vi "ROI Stand alone - get previous Zstack protocol.vi"(8 "error in (no error)":errorcluster, 11 "path":path) -> (0 "error out":errorcluster, 1 "Protocol":string, 2 "Frame Size":T1=200 items=["100X100"=100, "128X128"=128, "200X200"=200, "256X256"=256, "512X512"=512, "1024x1024"=1024, "2048x2048"=2048], 3 "field of view":dbl, 5 "zoom":dbl)   [LabVIEW 2020]
uses:
  Typedefs/Frame Size.ctl
  Visualisation/Functional Imaging Viewer/SubVIs/Experiment header interface/Typedefs/Header file actions.ctl
  Visualisation/Functional Imaging Viewer/SubVIs/Experiment header interface/Typedefs/Header file sections.ctl
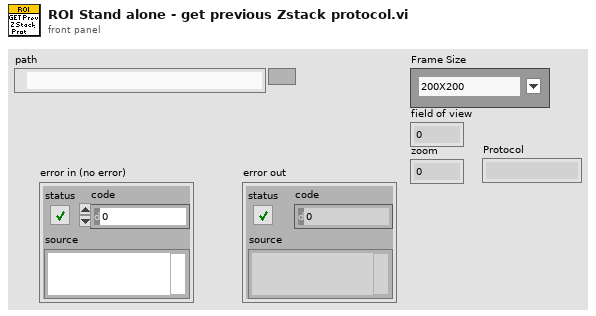
[diagram p1: front panel]
types:
  T1 = typedef "Frame Size.ctl" = u16
  T2 = typedef "Header file sections.ctl" = enum16{"ALL SECTIONS", "LOGIN", "GLOBAL PARAMETERS", "CALIBRATION DATA", "IMAGING MODES", "TIME SERIES", "MOTOR Z-STACK", "AOL Z-STACK", "FUNCTIONAL IMAGING", "VOLUME IMAGING", "MOVEMENT CORRECTION", "CALIBRATION", "STATISTICS", "BIOLOGY INFORMATION"}
  T3 = typedef "Header file actions.ctl" = enum16{"Create", "Open", "Read All", "Read Section", "Write All", "Write Section", "Close"}
  T4 = typedef "Header parameters cluster-ALL.ctl" = cluster{"LOGIN":T5, "GLOBAL PARAMETERS":T6, "IMAGING MODES":T8, "TIME SERIES":T9, "MOTOR Z-STACK ":T11, "AOL Z-STACK":T12, "FUNCTIONAL IMAGING":T13, "VOLUME IMAGING":T13, "MOVEMENT CORRECTION":T17, "CALIBRATION":T19, "STATISTICS":T20, "BIOLOGY INFORMATION":T21, "Calibration Data":T22}
  T5 = typedef "Header params -Login.ctl" = cluster{"User":string, "Profile":string, "Software Version":string, "Experiment Date Time":timestamp}
  T6 = typedef "Header params-Global Parameters.ctl" = cluster{"MicroscopeID":string, "Microscope Type":string, "Objective":string, "Field of View (um)":dbl, "Fill time (us)":dbl, "Experiment Type":T7, "Stimuli Trigger":bool, "Speed Logging":bool}
  T7 = typedef "Experiment Type.ctl" = enum16{"In vivo", "In vitro", "Testing", "Calibration", "Other"}
  T8 = typedef "Header params-Imaging Modes.ctl" = cluster{"Time Series":bool, "Motor Zstack":bool, "AOL Zstack":bool, "Functional Imaging":bool, "Volume Imaging":bool}
  T9 = typedef "Header params-Time Series.ctl" = cluster{"Basic Image meta data":T10, "AOL z":dbl}
  T10 = typedef "Header params-Basic image meta data.ctl" = cluster{"Wavelength (nm)":dbl, "# averaged frames":dbl, "laser power (%)":dbl, "Pockels":dbl, "pixel dwell time (us)":dbl, "pmt 1":dbl, "pmt 2":dbl, "back apperture":dbl, "zoom":dbl, "field of view":dbl, "Frame Size":T1, "AOL x centre":dbl, "AOL y centre":dbl, "Stage x position":dbl, "Stage y position":dbl, "Stage z position":dbl}
  T11 = typedef "Header params-Motor Z-stack.ctl" = cluster{"Hdr Basic Image meta data":T10, "Z Start":dbl, "Z Stop":dbl, "No of Planes":i32, "Laser Power (%) at Z Start":dbl, "Laser Power (%) at Z Stop":dbl}
  T12 = typedef "Header params-AOL Z-stack.ctl" = cluster{"Hdr Basic Image meta data":T10, "Z Start":dbl, "Z Stop":dbl, "No of Planes":i32, "Laser Power (%) at Z Start":dbl, "Laser Power (%) at Z Stop":dbl}
  T13 = typedef "Header params-Functional Imaging.ctl" = cluster{"Functional Mode":T14, "Variable Length":bool, "Variable Resolution":bool, "Pockels Modulation":bool, "Stimuli Trigger":bool, "Cool down enabled":bool, "AOL Mode":T15, "Plane Mode":T16, "Miniscan Dwell time per pixel (us)":dbl, "poi dwell time":dbl, "Number of trials":dbl, "Number of cycles":dbl, "Number of pois":dbl, "Number of miniscans":dbl, "Number of pixels in miniscan":dbl, "Rectangle ROI length":dbl, "Rectangle ROI height":dbl, "Frame rate (fps)":dbl, "Acquisition Length":dbl, "video length (sec)":dbl, "Stimuli delay (sec)":dbl, "Cool down time (sec)":dbl, "Basic Image meta data":T10, "Z Start (um)":dbl, "Z Stop (um)":dbl}
  T14 = typedef "Functional Mode.ctl" = enum16{"Point", "Line", "Patch", "Plane", "Volume"}
  T15 = typedef "AOL modes.ctl" = enum16{"Raster", "Structural", "Pointing", "Mini Scan", "Alignment"}
  T16 = typedef "Plane Mode.ctl" = u16
  T17 = typedef "Header params-Movement correction.ctl" = cluster{"Movement Correction":bool, "Axial Reference":bool, "Reference Source":T18, "Full Frame Size":dbl, "Reference Field of View":dbl, "Reference Zoom":dbl, "Reference dwell time (us)":dbl, "Reference X Pixels":dbl, "Reference Y Pixels":dbl, "Number of Z lines":dbl, "Size of Z pixels":dbl, "Axial Pixels":dbl, "Ignore Z lines":dbl, "Reference Scan Cycles":dbl, "Reference Threshold XY":dbl, "Reference Threshold Z":dbl, "Reference Average XY":dbl, "Reference Average Z":dbl, "Proportional Scale":dbl, "Integral Scale":dbl, "Proportional Scale Z":dbl, "Integral Scale Z":dbl, "Diff Threshold":dbl, "Diff Threshold Z":dbl, "Sliding Average":bool, "Reference count reset enabled":bool, "Scan Interval (ms)":dbl, "Ref Plot Refresh Rate (ms)":dbl}
  T18 = typedef "Reference source.ctl" = enum16{"Green channel", "Red channel"}
  T19 = typedef "Header params-Calibration Setup.ctl" = cluster{"Pockels Calibration File":path, "Calibration_ini file":path, "Setup_ini file":path}
  T20 = typedef "Header params-statistics.ctl" = cluster{"Z-stack duration (sec)":dbl, "Number of acquired data-points":dbl, "Acquisition time (ms)":dbl, "Number of acquired frames":dbl, "Intertrial times":dbl[]}
  T21 = typedef "Biology Information.ctl" = cluster{"Animal Code or Name":string, "Animal DoB":string, "Animal Age":string, "Animal Sex":string, "Animal Weight":string, "Date of Injection":string, "Date of Implant":string, "Site of Injection":string, "Animal Ear Notch":string, "AAV constructs":string, "Genetic background":string, "Optical reporter":string, "Region of brain imaged":string, "Other \ncomments":string}
  T22 = typedef "Header params-calibration data.ctl" = cluster{"Objective Name":string, "Calibration Wavelength":dbl, "Sum X":dbl, "Sum Y":dbl, "Diff X":dbl, "Diff Y":dbl, "Distortion Correction":dbl, " Z norm to um Scaling":dbl, " X norm to um Scaling":dbl}
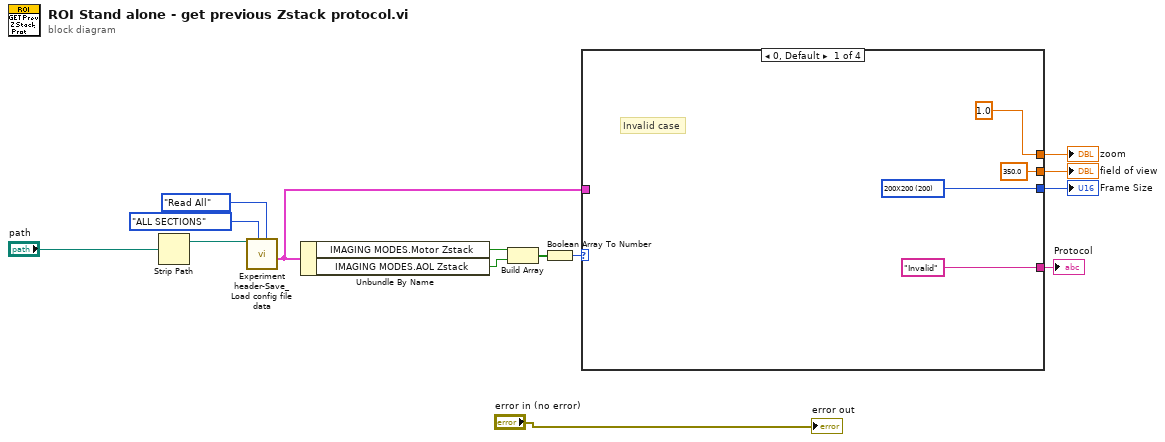
[diagram p0: block diagram]
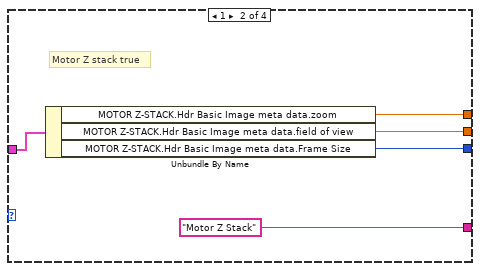
[diagram p2: hidden frame]
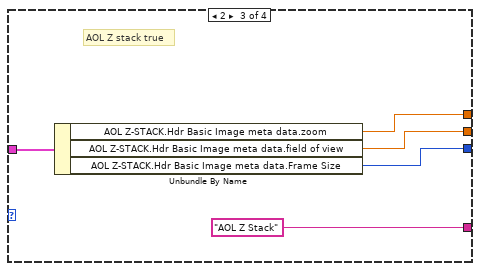
[diagram p3: hidden frame]
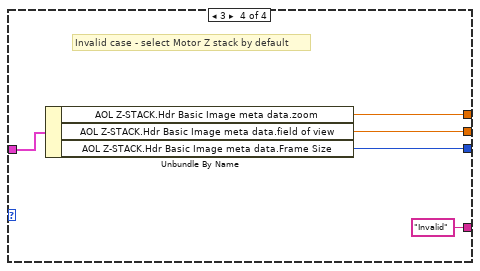
[diagram p4: hidden frame]
diagram:
  n1 = Strip Path(path="path") -> (stripped path=w14:path)  [unwired: 1 out]
  n2 = call "Experiment header-Save_Load config file data.vi"("Header file actions"=Header_file_actions."Read All", "Header file sections"=Header_file_sections."ALL SECTIONS", "Experiment data folder path"=w14) -> ("All header parameters out"=w6:T4)  [unwired: 7 in, 1 out]
  n3 = Unbundle By Name(w6) -> ("IMAGING MODES.Motor Zstack"=w10:bool, "IMAGING MODES.AOL Zstack"=w9:bool)
  n4 = Build Array(w10, w9) -> (w8:bool[])
  n5 = Boolean Array To Number(Boolean array=w8) -> (number=w7:u32)
  n6 = case shown="0, Default" w7 {
    tunnel: w6 -> [_ w23 w27 w33]
    tunnel: [w18 w22 w24 w32] -> w5
    tunnel: ["Invalid" "Motor Z Stack" "AOL Z Stack" "Invalid"] -> w4
    tunnel: [1.0 ("zoom") w19 w26 w30] -> w1
    tunnel: [350.0 ("field of view") w20 w25 w29] -> w2
    frame 0, Default {
      w18 = T1 200 items=["100X100"=100, "128X128"=128, "200X200"=200, "256X256"=256, "512X512"=512, "1024x1024"=1024, "2048x2048"=2048] ("Frame Size")
      # "Invalid case"
    }
    frame 1 {
      # "Motor Z stack true"
      n7 = Unbundle By Name(w23) -> ("MOTOR Z-STACK.Hdr Basic Image meta data.zoom"=w19:dbl, "MOTOR Z-STACK.Hdr Basic Image meta data.field of view"=w20:dbl, "MOTOR Z-STACK.Hdr Basic Image meta data.Frame Size"=w22:T1)
    }
    frame 2 {
      # "AOL Z stack true"
      n8 = Unbundle By Name(w27) -> ("AOL Z-STACK.Hdr Basic Image meta data.zoom"=w26:dbl, "AOL Z-STACK.Hdr Basic Image meta data.field of view"=w25:dbl, "AOL Z-STACK.Hdr Basic Image meta data.Frame Size"=w24:T1)
    }
    frame 3 {
      # "Invalid case - select Motor Z stack by default"
      n9 = Unbundle By Name(w33) -> ("AOL Z-STACK.Hdr Basic Image meta data.zoom"=w30:dbl, "AOL Z-STACK.Hdr Basic Image meta data.field of view"=w29:dbl, "AOL Z-STACK.Hdr Basic Image meta data.Frame Size"=w32:T1)
    }
  }
  "Frame Size" <- w5
  "Protocol" <- w4
  "field of view" <- w2
  "zoom" <- w1
  "error out" <- "error in (no error)"
